vi "SE FP hindbrain THINK.vi"(5 "error in":errorcluster, 6 "BLUE LED":bool=TRUE, 7 "Forebrain Comd":T2, 8 "RUN?":bool=TRUE, 9 "MANUAL":bool=TRUE, 10 "GREEN LED":bool=TRUE, 11 "RED LED":bool=TRUE) -> (0 "error out":errorcluster, 1 "BLUE LED OUT":bool=TRUE, 2 "GREEN LED OUT":bool=TRUE, 3 "LED array":bool[](array[boolean]), 4 "RED LED OUT":bool=TRUE)   [LabVIEW 2014]
doc: "This vi is the THINK portion of the Hindbrain...at present it has not function and is a place holder for later development."
panel:
  in  "Boat Status":T1={"GPS"={"X pos"=0, "Y pos"=0, "Heading"=0.0}, "IR Sensors"=[{"Name"="Bow", "Angle"=0.0, "Distance"=0.0}], "MOT BAT"=7.2, "RIO BAT"=7.2}
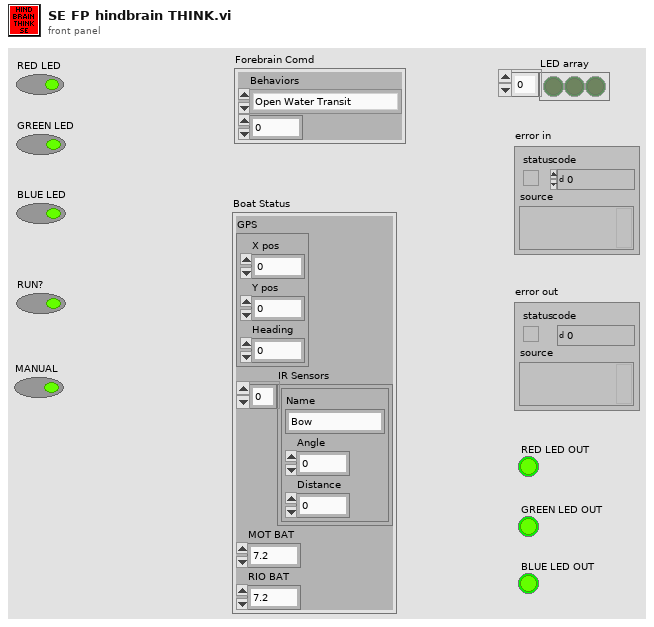
[diagram p1: front panel]
types:
  T1 = cluster{"GPS":cluster{"X pos":i32, "Y pos":i32, "Heading":dbl}, "IR Sensors":cluster{"Name":string, "Angle":dbl, "Distance":dbl}[], "MOT BAT":dbl, "RIO BAT":dbl}
  T2 = cluster{"Behaviors":enum16{"Open Water Transit", "P-Wall Follow", "S-Wall Follow", "Dock"}, dbl}
  T3 = enum16{"Open Water Transit", "P-Wall Follow", "S-Wall Follow", "Dock"}
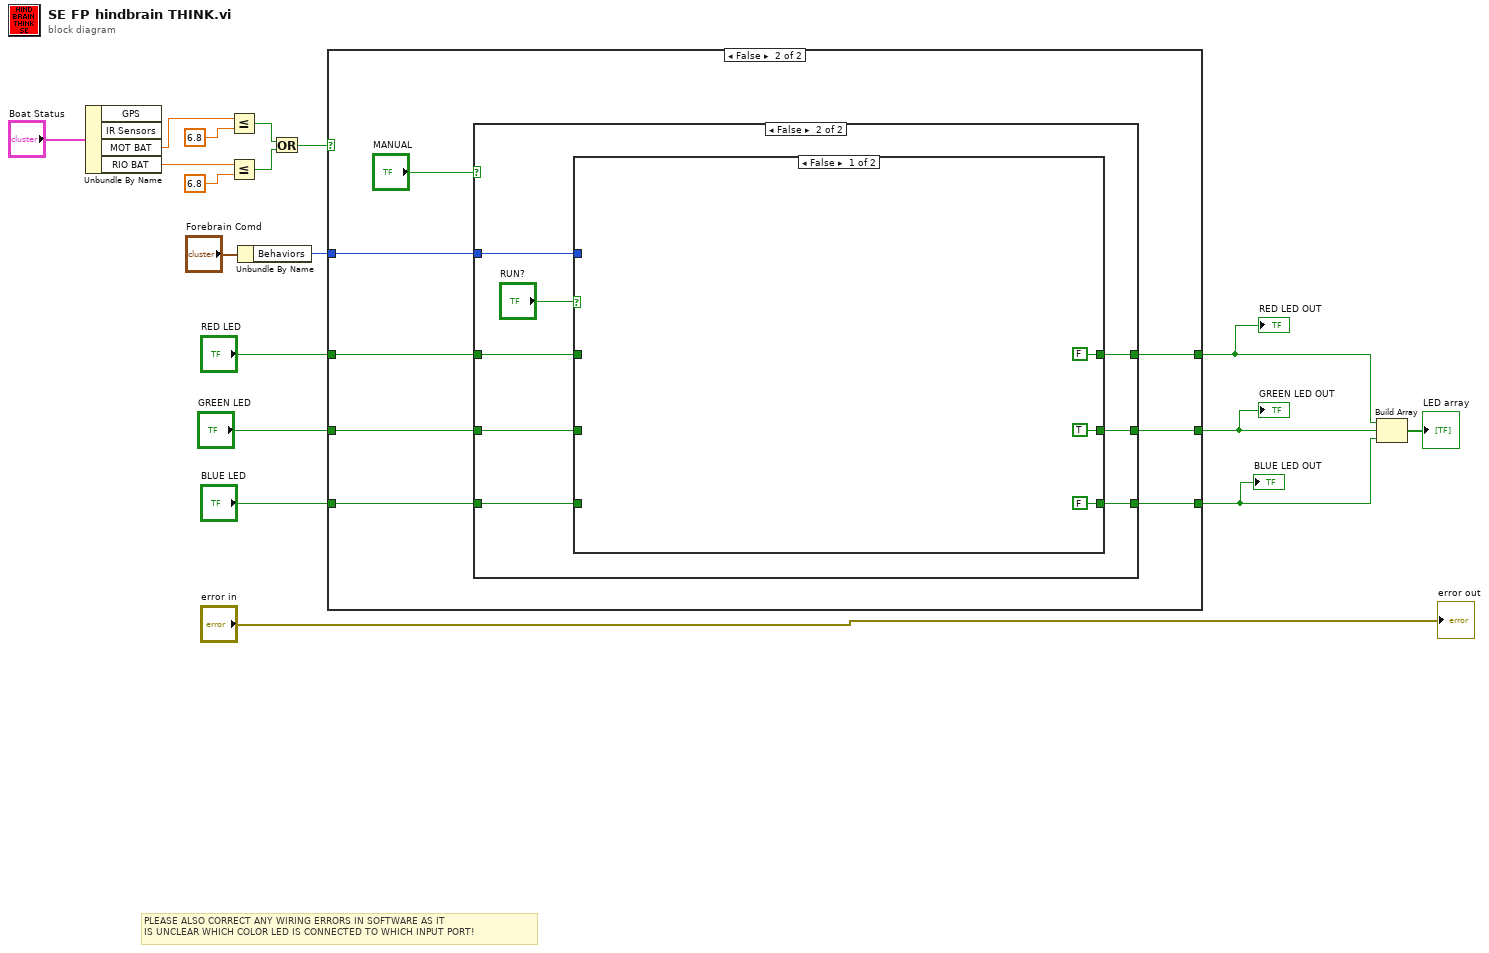
[diagram p0: block diagram]
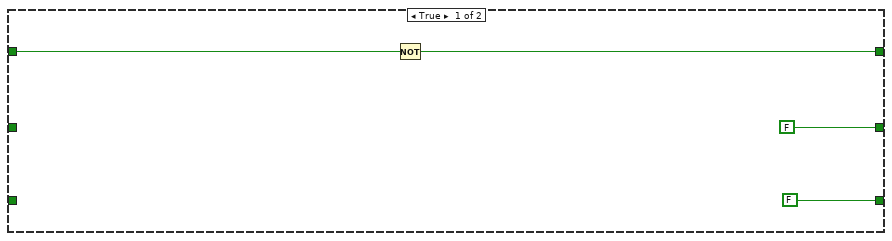
[diagram p2: hidden frame]
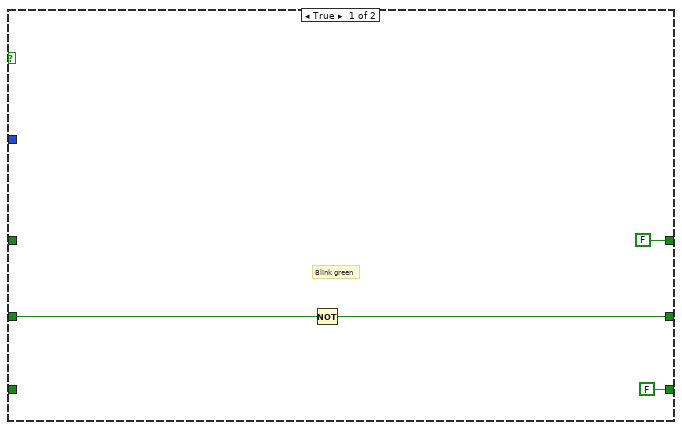
[diagram p3: hidden frame]
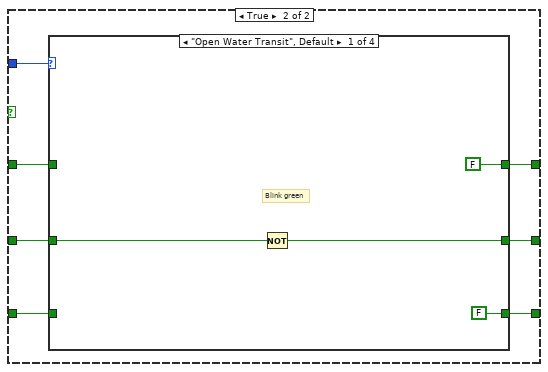
[diagram p4: hidden frame]
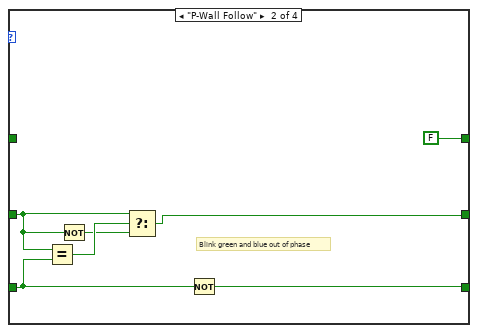
[diagram p5: hidden frame]
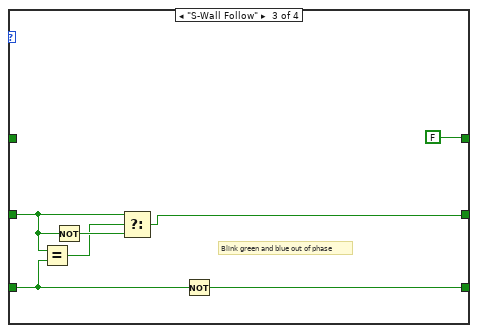
[diagram p6: hidden frame]
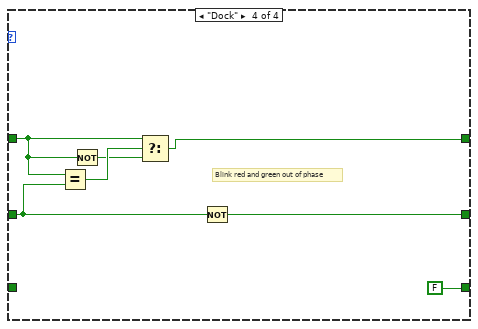
[diagram p7: hidden frame]
diagram:
  # "PLEASE ALSO CORRECT ANY WIRING ERRORS IN SOFTWARE AS IT\nIS UNCLEAR WHICH COLOR LED IS CONNECTED TO WHICH INPUT PORT!"
  n1 = Unbundle By Name("Boat Status") -> ("MOT BAT"=w9:dbl, "RIO BAT"=w8:dbl)  [unwired: 2 out]
  n2 = Less Or Equal?(x=w9, y=6.8) -> (x <= y?=w7:bool)
  n3 = Less Or Equal?(x=w8, y=6.8) -> (x <= y?=w6:bool)
  n4 = Unbundle By Name("Forebrain Comd") -> ("Behaviors"=w13:T3)
  n5 = Or(x=w7, y=w6) -> (x .or. y?=w5:bool)
  n6 = case shown="False" w5 {
    tunnel: "RED LED" -> [w22 w30]
    tunnel: "GREEN LED" -> [_ w29]
    tunnel: "BLUE LED" -> [_ w28]
    tunnel: w13 -> [_ w27]
    tunnel: [w21 w26] -> w3
    tunnel: [FALSE w25] -> w4
    tunnel: [FALSE w24] -> w2
    frame True {
      n7 = Not(x=w22) -> (.not. x?=w21:bool)
    }
    frame False {
      n8 = case shown="False" "MANUAL" {
        tunnel: w30 -> [_ w42]
        tunnel: w29 -> [w34 w41]
        tunnel: w28 -> [_ w40]
        tunnel: w27 -> [_ w39]
        tunnel: [FALSE w38] -> w26
        tunnel: [w33 w37] -> w25
        tunnel: [FALSE w36] -> w24
        frame True {
          # "Blink green"
          n9 = Not(x=w34) -> (.not. x?=w33:bool)
        }
        frame False {
          n10 = case shown="False" "RUN?" {
            tunnel: w42 -> [_ w52]
            tunnel: w41 -> [_ w51]
            tunnel: w40 -> [_ w50]
            tunnel: w39 -> [_ w49]
            tunnel: [FALSE ("RED LED") w48] -> w38
            tunnel: [TRUE ("GREEN LED") w47] -> w37
            tunnel: [FALSE w46] -> w36
            frame False {
            }
            frame True {
              n11 = case shown="\"Open Water Transit\", Default" w49 {
                tunnel: w52 -> [_ _ _ w74]
                tunnel: w51 -> [w56 w58 w64 w73]
                tunnel: w50 -> [_ w61 w65 _]
                tunnel: [FALSE FALSE FALSE w75] -> w48
                tunnel: [w55 w57 w68 w72] -> w47
                tunnel: [FALSE w60 w67 FALSE] -> w46
                frame "Open Water Transit", Default {
                  # "Blink green"
                  n12 = Not(x=w56) -> (.not. x?=w55:bool)
                }
                frame "P-Wall Follow" {
                  # "Blink green and blue out of phase"
                  n13 = Equal?(x=w58, y=w61) -> (x = y?=w62:bool)
                  n14 = Not(x=w58) -> (.not. x?=w59:bool)
                  n15 = Select(t=w58, s=w62, f=w59) -> (s? t:f=w57:bool)
                  n16 = Not(x=w61) -> (.not. x?=w60:bool)
                }
                frame "S-Wall Follow" {
                  # "Blink green and blue out of phase"
                  n17 = Equal?(x=w64, y=w65) -> (x = y?=w69:bool)
                  n18 = Not(x=w64) -> (.not. x?=w70:bool)
                  n19 = Select(t=w64, s=w69, f=w70) -> (s? t:f=w68:bool)
                  n20 = Not(x=w65) -> (.not. x?=w67:bool)
                }
                frame "Dock" {
                  # "Blink red and green out of phase"
                  n21 = Equal?(x=w74, y=w73) -> (x = y?=w77:bool)
                  n22 = Not(x=w74) -> (.not. x?=w76:bool)
                  n23 = Select(t=w74, s=w77, f=w76) -> (s? t:f=w75:bool)
                  n24 = Not(x=w73) -> (.not. x?=w72:bool)
                }
              }
            }
          }
        }
      }
    }
  }
  "BLUE LED OUT" <- w2
  "RED LED OUT" <- w3
  "GREEN LED OUT" <- w4
  n25 = Build Array(w3, w4, w2) -> (→"LED array":bool[])
  "error out" <- "error in"
